vi "Configure Hardware_original.vi"() -> ()   [LabVIEW 2017]
uses:
  5c499f86-0740-4f3d-9c1c-78667029dad4.vi
panel:
  in  "DMM":i32(listbox)
  in  "Signal Generator 2":i32(listbox)
  in  "Oscilloscope 2":i32(listbox)=1
  in  "Signal Generator":i32(listbox)
  in  "Oscilloscope":i32(listbox)=1
  # "Configure Hardware"
  # "Select Your Hardware"
  # "Select Your Hardware"
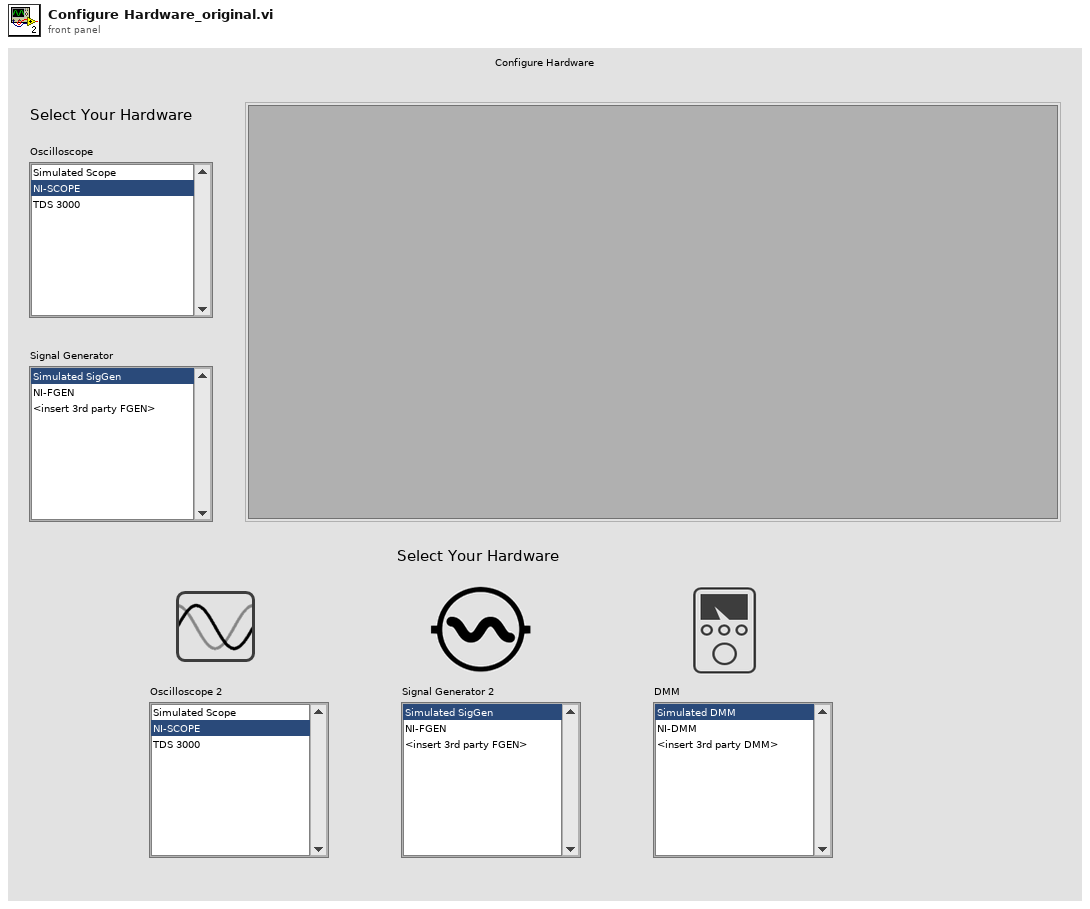
[diagram p1: front panel]
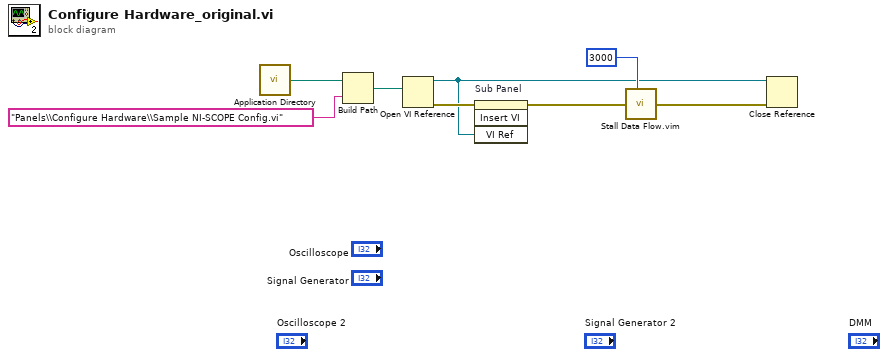
[diagram p0: block diagram]
diagram:
  n1 = call <vilib>:"Application Directory.vi"() -> ("Application Directory"=w8:path)
  n2 = Build Path(base path=w8, name or relative path="Panels\\Configure Hardware\\Sample NI-SCOPE Config.vi") -> (appended path=w6:path)
  n3 = Open VI Reference(vi path=w6) -> (vi reference=w1:refnum<vi>, error out=w5:errorcluster)  [unwired: 5 in]
  n4 = invoke on="Sub Panel" class="SubPnl" method="Insert VI"(error in=w5, "VI Ref"=w1) -> (error out=w4:errorcluster)  [unwired: 2 in, 3 out]
  n5 = call "Stall Data Flow.vim"("value in"=w4, "milliseconds to wait"=u32 3000) -> ("value out"=w3:errorcluster)  [unwired: 1 out]
  n6 = Close Reference(reference=w1, error in (no error)=w3) -> ()  [unwired: 1 out]
